vi "maze_v2.5.vi"   [LabVIEW 2012]
uses:
  <vilib>/NXT/Subs/MotorOutput.ctl
  <vilib>/NXT/Block Support/NXT_InputPort.ctl
  <vilib>/NXT/Dual Mode Library/Motors/MotorReverse.vi
  <vilib>/NXT/Dual Mode Library/Motors/MotorOn.vi
  <vilib>/NXT/Dual Mode Library/Motors/MotorBrake.vi
  <vilib>/NXT/Dual Mode Library/Display/clearDisplay.vi
  <vilib>/NXT/Dual Mode Library/Display/drawText.vi
  <vilib>/NXT/Dual Mode Library/Waits/Wait_Num(msec).vi
  <vilib>/NXT/Dual Mode Library/Display/drawLine.vi
  <vilib>/NXT/Dual Mode Library/Waits/Wait_Num.vi
  <vilib>/NXT/Dual Mode Library/Display/drawNumber.vi
types:
  T1 = typedef "MotorOutput.ctl" = u8
  T2 = typedef "LVHSConnector.ctl" = cluster{"Hardware":string, "Flattened String":string}
  T3 = typedef "NXT_InputPort.ctl" = u8
  T4 = cluster{"x":i32, "Start X":i16, "x":i32, "Start X":i16}
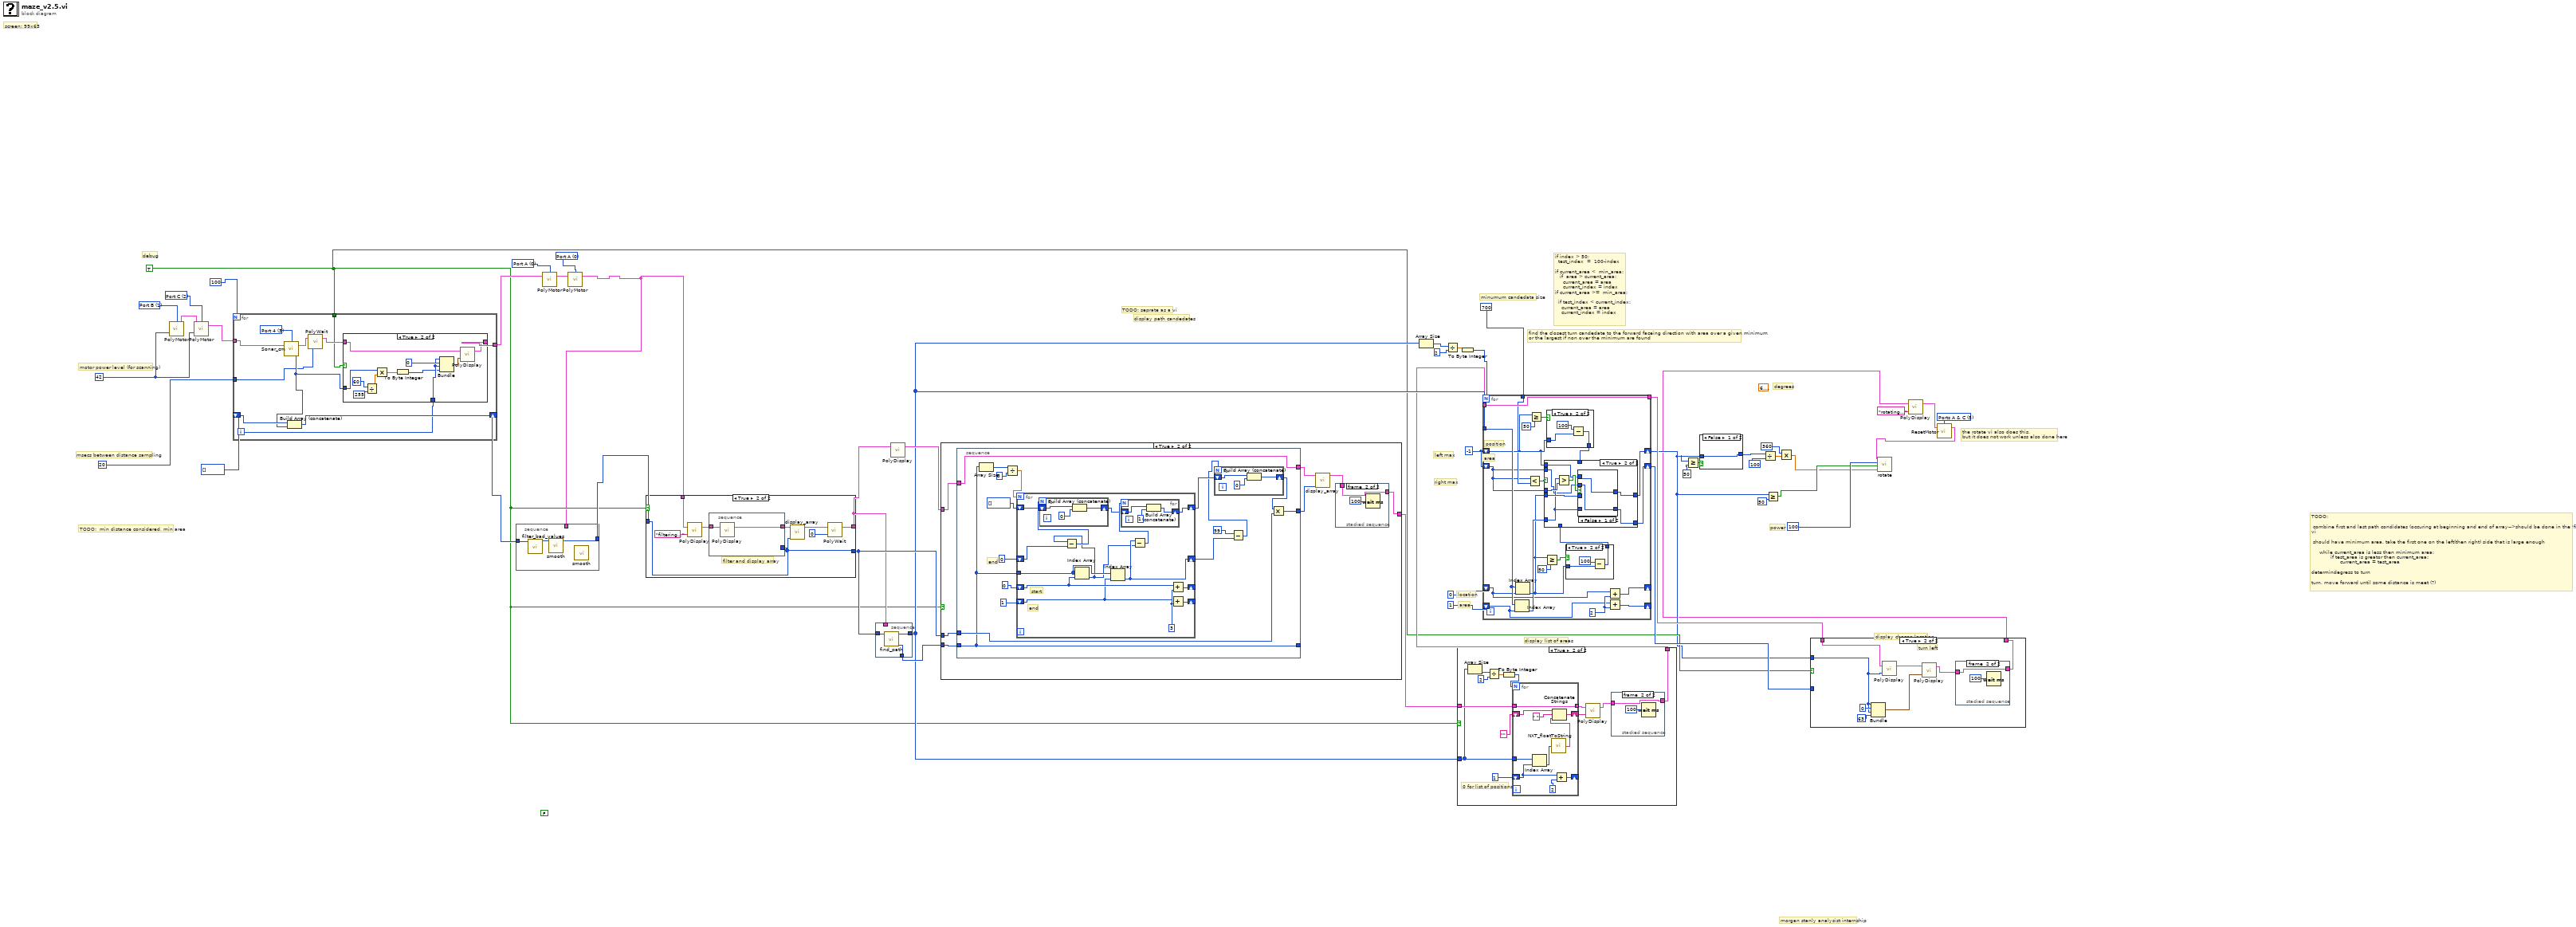
[diagram p0: block diagram]
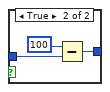
[diagram p2: hidden frame]
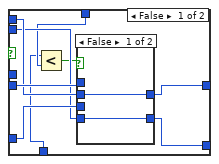
[diagram p8: hidden frame]
diagram:
  w5 = T1 5 items=["Port A"=0, "Port B"=1, "Port C"=2, "Ports A & B"=4, "Ports A & C"=5, "Ports B & C"=6, "All Ports"=3] ("Port (All Ports)")
  (unwired) 6.283185307179586 ("Pi Multiplied By 2")
  w21 = i16 -1 ("Start X")
  w38 = T1 0 items=["Port A"=0, "Port B"=1, "Port C"=2, "Ports A & B"=4, "Ports A & C"=5, "Ports B & C"=6, "as"=3] ("Output Port (All Ports)")
  w40 = T1 0 items=["Port A"=0, "Port B"=1, "Port C"=2, "Ports A & B"=4, "Ports A & C"=5, "Ports B & C"=6, "as"=3] ("Output Port (All Ports)")
  (unwired) FALSE
  w19 = TRUE
  w45 = 42 ("Power (75)")
  w47 = T1 2 items=["Port A"=0, "Port B"=1, "Port C"=2, "Ports A & B"=4, "Ports A & C"=5, "Ports B & C"=6, "as"=3] ("Output Port (All Ports)")
  w49 = T1 1 items=["Port A"=0, "Port B"=1, "Port C"=2, "Ports A & B"=4, "Ports A & C"=5, "Ports B & C"=6, "as"=3] ("Output Port (All Ports)")
  # "the rotate vi also does this,\nbut it does not work unless also done here"
  # "power"
  # "degrees"
  # "display chosen location"
  # "display list of areas"
  # "if index > 50;\n  test_index  =  100-index\n\nif current_area <  min_area:\n   if  area > current_area:\n     current_area = area\n     current_index = index\nif current_area >=  min_area:\n\n  if test_index < current_index:\n    current_area = area\n    current_index = index"
  # "morgan stanly analysist internship"
  # "minumum candedata size"
  # "find the closest turn candedate to the forward faceing direction with area over a given minimum\nor the largest if non over the minimum are found"
  # "TODO:  min distance considered, min area"
  # "msecs between distance sampling"
  # "motor power level (for scanning)"
  # "TODO: seprate as a vi"
  # "TODO:\n\n combine first and last path condidates (occuring at beginning and end of array-->should be done in the 'find paths' vi\n            \n should have minimum area, take the first one on the left(then right) side that is large enough\n\n     while current_area is less then minimum area:\n            if test_area is greator then current_area:\n                  current_area = test_area\n\ndetermindegress to turn\n\nturn, move forward until some distance is meet (?)"
  # "right max"
  # "left max"
  # "display path candedates"
  # "area"
  # "location"
  # "debug"
  # "screen: 99x63"
  n1 = call-poly <vilib>:"PolyMotor.vi"("Power (75)"=w45, "Output Port (All Ports)"=w49) -> ("NXT"=w48:T2)  [unwired: 2 in]
  n2 = call-poly <vilib>:"PolyMotor.vi"("Power (75)"=w45, "NXT"=w48, "Output Port (All Ports)"=w47) -> ("NXT"=w46:T2)  [unwired: 1 in]
  n3 = for {
    N: 100 -> [_]
    shift-right: [w57] -> w42
    shift-left: i16[] [] -> [w58]
    tunnel: w46 -> [w60]
    tunnel: [w54] -> w39
    tunnel: w19 -> [w53]
    tunnel: 20 -> [w50]
    i -> [w51]
    w59 = T3 3 items=["Port 1", "Port 2", "Port 3", "Port 4"] ("Port (Port 4)")
    n4 = call <vilib>:"Sonar_cm.vi"("NXT"=w60, "Port (Port 4)"=w59) -> ("Distance (cm)"=w52:i16, "NXT"=w56:T2)  [unwired: 1 in]
    n5 = Build Array (concatenate)(w58, w52) -> (w57:i16[])
    n6 = call-poly <vilib>:"PolyWait.vi"("Time (100 msec)"=w50, "NXT"=w56) -> ("NXT"=w55:T2)  [unwired: 2 in]
    n7 = case shown="True" w53 {
      tunnel: w55 -> [w61 w69]
      tunnel: [w61 w70] -> w54
      tunnel: w52 -> [_ w68]
      tunnel: w51 -> [_ w63]
      frame False {
      }
      frame True {
        n8 = Divide(x=i16 60 ("Start X"), y=i16 255 ("Start X")) -> (x/y=w66:dbl)
        n9 = Multiply(x=w68, y=w66) -> (x*y=w71:dbl)
        n10 = To Byte Integer(number=w71) -> (8bit integer=w62:i8)
        n11 = Bundle(w63, "Start X"=i16 0, w63, w62) -> (w64:cluster{i32, "Start X":i16, i32, i8})  [unwired: 1 in]
        n12 = call-poly <vilib>:"PolyDisplay.vi"("Line Parameters"=w64, "NXT"=w69) -> ("NXT"=w70:T2)  [unwired: 2 in]
      }
    }
  }
  n13 = call-poly <vilib>:"PolyMotor.vi"("NXT"=w39, "Port (All Ports)"=w40) -> ("NXT"=w41:T2)  [unwired: 2 in]
  n14 = call-poly <vilib>:"PolyMotor.vi"("NXT"=w41, "Port (All Ports)"=w38) -> ("NXT"=w1:T2)  [unwired: 2 in]
  n15 = stacked-sequence {
    tunnel: w42 -> [w74]
    tunnel: [w73] -> w37
    tunnel: w1 -> [_]
    frame #0 {
      n16 = call "filter_bad_values.vi"("Array 3"=w74) -> ("Array 4"=w75:i32[])  [unwired: 10 in]
      n17 = call "smooth.vi"("Array"=w75) -> ("Array 2"=w73:i32[])  [unwired: 10 in]
      n18 = call "smooth.vi"() -> ()  [unwired: 11 in, 1 out]
    }
  }
  n19 = case shown="True" w19 {
    tunnel: w1 -> [w77 w82]
    tunnel: w37 -> [w76 w78]
    tunnel: [w77 w79] -> w34
    tunnel: [w76 w78] -> w36
    frame False {
    }
    frame True {
      # "filter and display array"
      n20 = call-poly <vilib>:"PolyDisplay.vi"("Text"="filtering...", "NXT"=w82) -> ("NXT"=w83:T2)  [unwired: 2 in]
      n21 = stacked-sequence {
        tunnel: [w87] -> w81
        tunnel: w78 -> [_]
        tunnel: w83 -> [w86]
        frame #0 {
          n22 = call-poly <vilib>:"PolyDisplay.vi"("NXT"=w86) -> ("NXT"=w87:T2)  [unwired: 3 in]
        }
      }
      n23 = call "display_array.vi"("array"=w78, "NXT"=w81) -> ("NXT 2"=w80:T2)  [unwired: 9 in]
      n24 = call-poly <vilib>:"PolyWait.vi"("Time (1 sec)"=i16 0 ("Start X"), "NXT"=w80) -> ("NXT"=w79:T2)  [unwired: 2 in]
    }
  }
  n25 = stacked-sequence {
    tunnel: w36 -> [w90]
    tunnel: [w89] -> w35
    tunnel: w34 -> [_]
    tunnel: [w88] -> w25
    frame #0 {
      n26 = call "find_path.vi"("Array"=w90) -> ("debug array"=w89:i32[], "Array 2"=w88:i32[])  [unwired: 9 in]
    }
  }
  n27 = call-poly <vilib>:"PolyDisplay.vi"("NXT"=w34) -> ("NXT"=w33:T2)  [unwired: 3 in]
  n28 = case shown="True" w19 {
    tunnel: w35 -> [_ w97]
    tunnel: w33 -> [w91 w96]
    tunnel: [w91 w93] -> w27
    tunnel: w36 -> [_ w98]
    frame False {
    }
    frame True {
      n29 = stacked-sequence {
        tunnel: w98 -> [w112]
        tunnel: [w111] -> w92
        tunnel: w97 -> [w101]
        tunnel: w96 -> [w102]
        tunnel: [w102] -> w95
        tunnel: [w101] -> _
        frame #0 {
          # "end"
          n30 = Array Size(array=w101) -> (size(s)=w105:i32)
          n31 = Divide(x=w105, y=3) -> (x/y=w103:dbl)
          n32 = for {
            N: w103 -> [_]
            shift-right: [w132] -> _
            shift-left: i16 0 ("Start X") -> [w129]
            shift-right: [w131] -> _
            shift-left: i16 1 ("Start X") -> [w128]
            shift-right: [w120] -> w110
            shift-left: i16[] [] -> [w122]
            tunnel: w101 -> [w127]
            shift-right: [w125] -> w107
            shift-left: i16 0 ("Start X") -> [w126]
            w133 = 3 ("y")
            # "end"
            # "start"
            n33 = Index Array(array=w127, index=w129) -> (element=w124:i32)
            n34 = Subtract(x=w124, y=w126) -> (x-y=w130:i32)
            n35 = for {
              N: w130 -> [_]
              shift-right: [w138] -> w121
              shift-left: w122 -> [w139]
              n36 = Build Array (concatenate)(w139, i16 0 ("Start X")) -> (w138:i16[])
            }
            n37 = Index Array(array=w127, index=w128) -> (element=w125:i32)
            n38 = Subtract(x=w125, y=w124) -> (x-y=w123:i32)
            n39 = for {
              N: w123 -> [_]
              shift-right: [w134] -> w120
              shift-left: w121 -> [w135]
              n40 = Build Array (concatenate)(w135, i16 1 ("Start X")) -> (w134:i16[])
            }
            n41 = Add(x=w129, y=w133) -> (x+y=w132:i32)
            n42 = Add(x=w128, y=w133) -> (x+y=w131:i32)
          }
          n43 = Subtract(x=i16 99 ("Start X"), y=w107) -> (x-y=w106:i32)
          n44 = for {
            N: w106 -> [_]
            shift-right: [w118] -> w109
            shift-left: w110 -> [w119]
            n45 = Build Array (concatenate)(w119, i16 0 ("Start X")) -> (w118:i16[])
          }
          n46 = Multiply(x=w109, y=w112) -> (x*y=w111:i32[])
        }
      }
      n47 = call "display_array.vi"("array"=w92, "NXT"=w95) -> ("NXT 2"=w94:T2)  [unwired: 9 in]
      n48 = stacked-sequence {
        tunnel: [_ w99] -> w93
        tunnel: w94 -> [_ w99]
        frame #0 {
        }
        frame #1 {
          n49 = Wait (ms)(milliseconds to wait=u32 100) -> ()  [unwired: 1 out]
        }
      }
    }
  }
  n50 = Array Size(array=w25) -> (size(s)=w30:i32)
  n51 = Divide(x=w30, y=2) -> (x/y=w28:dbl)
  n52 = case shown="True" w19 {
    tunnel: w27 -> [w140 w149]
    tunnel: w25 -> [_ w143]
    tunnel: [w140 w142] -> w24
    frame False {
    }
    frame True {
      # "0 for list of positions"
      n53 = Array Size(array=w143) -> (size(s)=w147:i32)
      n54 = Divide(x=w147, y=2) -> (x/y=w145:dbl)
      n55 = To Byte Integer(number=w145) -> (8bit integer=w144:i8)
      n56 = for {
        N: w144 -> [_]
        tunnel: w149 -> [w161]
        tunnel: [w161] -> w151
        shift-right: [w162] -> w150
        shift-left: "" ("Text") -> [w164]
        shift-right: [w159] -> _
        shift-left: i16 1 ("Start X") -> [w157]
        tunnel: w143 -> [w156]
        n57 = Index Array(array=w156, index=w157) -> (element=w155:i32)
        n58 = call <vilib>:"NXT_floatToString.vi"("number"=w155) -> ("string"=w163:string)
        n59 = Concatenate Strings(w164, " " ("Text"), w163) -> (w162:string)
        n60 = Add(x=w157, y=i16 2 ("Start X")) -> (x+y=w159:i16)
      }
      n61 = call-poly <vilib>:"PolyDisplay.vi"("Text"=w150, "NXT"=w151) -> ("NXT"=w141:T2)  [unwired: 2 in]
      n62 = stacked-sequence {
        tunnel: w141 -> [_ w153]
        tunnel: [_ w153] -> w142
        frame #0 {
        }
        frame #1 {
          n63 = Wait (ms)(milliseconds to wait=u32 100) -> ()  [unwired: 1 out]
        }
      }
    }
  }
  n64 = To Byte Integer(number=w28) -> (8bit integer=w26:i8)
  n65 = for {
    N: w26 -> [_]
    tunnel: w25 -> [w185]
    shift-right: [w184] -> _
    shift-left: i16 0 ("Start X") -> [w165]
    shift-right: [w183] -> _
    shift-left: i16 1 ("Start X") -> [w181]
    shift-right: [w175] -> w9
    shift-left: w21 -> [w169]
    shift-right: [w174] -> w20
    shift-left: w21 -> [w166]
    tunnel: w24 -> [w180]
    tunnel: i16 700 ("Start X") -> [w167]
    tunnel: [w180] -> w14
    w182 = i16 2 ("Start X")
    # "area"
    # "position"
    n66 = Index Array(array=w185, index=w181) -> (element=w176:i32)
    n67 = Index Array(array=w185, index=w165) -> (element=w168:i32)
    n68 = Less?(x=w166, y=w167) -> (x < y?=w177:bool)
    n69 = Greater Or Equal?(x=w169, y=i16 50 ("Start X")) -> (x >= y?=w178:bool)
    n70 = Greater Or Equal?(x=w168, y=i16 50 ("Start X")) -> (x >= y?=w172:bool)
    n71 = case shown="True" w178 {
      tunnel: w169 -> [w215 w216]
      tunnel: [w215 w218] -> w173
      frame False {
      }
      frame True {
        n72 = Subtract(x=i16 100 ("Start X"), y=w216) -> (x-y=w218:i32)
      }
    }
    n73 = case shown="True" w172 {
      tunnel: w168 -> [w186 w188]
      tunnel: [w186 w187] -> w170
      frame False {
      }
      frame True {
        n74 = Subtract(x=i16 100 ("Start X"), y=w188) -> (x-y=w187:i32)
      }
    }
    n75 = case shown="True" w177 {
      tunnel: w168 -> [w198 w208]
      tunnel: w176 -> [w197 w206]
      tunnel: [w196 w207] -> w175
      tunnel: [w195 w205] -> w174
      tunnel: w173 -> [w192 _]
      tunnel: w170 -> [w191 _]
      tunnel: w169 -> [w194 w204]
      tunnel: w166 -> [w193 w203]
      tunnel: w166 -> [_ w210]
      frame False {
        n76 = Less?(x=w191, y=w192) -> (x < y?=w190:bool)
        n77 = case shown="False" w190 {
          tunnel: w198 -> [_ w202]
          tunnel: w197 -> [_ w201]
          tunnel: [w200 w202] -> w196
          tunnel: [w199 w201] -> w195
          tunnel: w194 -> [w200 _]
          tunnel: w193 -> [w199 _]
          frame False {
          }
          frame True {
          }
        }
      }
      frame True {
        n78 = Greater?(x=w206, y=w210) -> (0:w209:bool)
        n79 = case shown="False" w209 {
          tunnel: w208 -> [_ w214]
          tunnel: [w211 w214] -> w207
          tunnel: w206 -> [_ w213]
          tunnel: [w212 w213] -> w205
          tunnel: w204 -> [w211 _]
          tunnel: w203 -> [w212 _]
          frame False {
          }
          frame True {
          }
        }
      }
    }
    n80 = Add(x=w165, y=w182) -> (x+y=w184:i16)
    n81 = Add(x=w181, y=w182) -> (x+y=w183:i16)
  }
  n82 = Greater Or Equal?(x=w9, y=i16 50 ("Start X")) -> (x >= y?=w11:bool)
  n83 = case shown="False" w11 {
    tunnel: w9 -> [w219 w220]
    tunnel: [w219 w222] -> w10
    frame False {
    }
    frame True {
      n84 = Subtract(x=i16 100 ("Start X"), y=w220) -> (x-y=w222:i32)
    }
  }
  n85 = Divide(x=w10, y=i16 100 ("Start X")) -> (x/y=w16:dbl)
  n86 = Greater Or Equal?(x=w9, y=i16 50 ("Start X")) -> (x >= y?=w8:bool)
  n87 = Multiply(x=i16 360 ("Start X"), y=w16) -> (x*y=w2:dbl)
  n88 = case shown="True" w19 {
    tunnel: w9 -> [_ w226]
    tunnel: w14 -> [w223 w228]
    tunnel: [w223 w224] -> w7
    tunnel: w20 -> [_ _]
    frame False {
      # "turn right"
    }
    frame True {
      # "turn left"
      n89 = Bundle("x"=w226, "Start X"=i16 0, "x"=w226, "Start X"=i16 63) -> (w227:T4)  [unwired: 1 in]
      n90 = call-poly <vilib>:"PolyDisplay.vi"("number"=w226, "NXT"=w228) -> ("NXT"=w231:T2)  [unwired: 2 in]
      n91 = call-poly <vilib>:"PolyDisplay.vi"("Line Parameters"=w227, "NXT"=w231) -> ("NXT"=w225:T2)  [unwired: 2 in]
      n92 = stacked-sequence {
        tunnel: w225 -> [_ w232]
        tunnel: [_ w232] -> w224
        frame #0 {
        }
        frame #1 {
          n93 = Wait (ms)(milliseconds to wait=u32 100) -> ()  [unwired: 1 out]
        }
      }
    }
  }
  n94 = call-poly <vilib>:"PolyDisplay.vi"("Text"="rotating...", "NXT"=w7) -> ("NXT"=w4:T2)  [unwired: 2 in]
  n95 = call <vilib>:"ResetMotor.vi"("NXT"=w4, "Port (All Ports)"=w5) -> ("NXT"=w3:T2)  [unwired: 2 in]
  n96 = call "rotate.vi"("degrees to  rotate"=w2, "right(T)/left(F)"=w8, "power"=u16 100 ("Max Value"), "NXT 2"=w3) -> ()  [unwired: 7 in, 1 out]
